vi "最大下移距离.vi"(9 "偏移量":cluster{"X":i32, "Y":i32}, 10 "数组 2":u32[][](array[colorbox]), 11 "数组":u32[][](array[colorbox])) -> (3 "最大下移距离":i32)   [LabVIEW 2012]
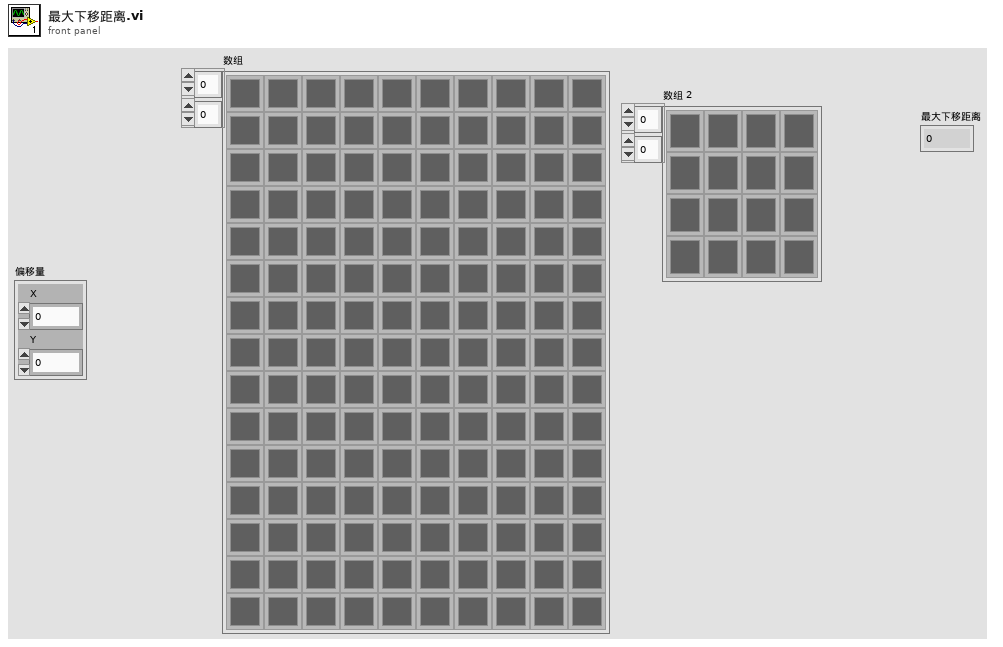
[diagram p1: front panel]
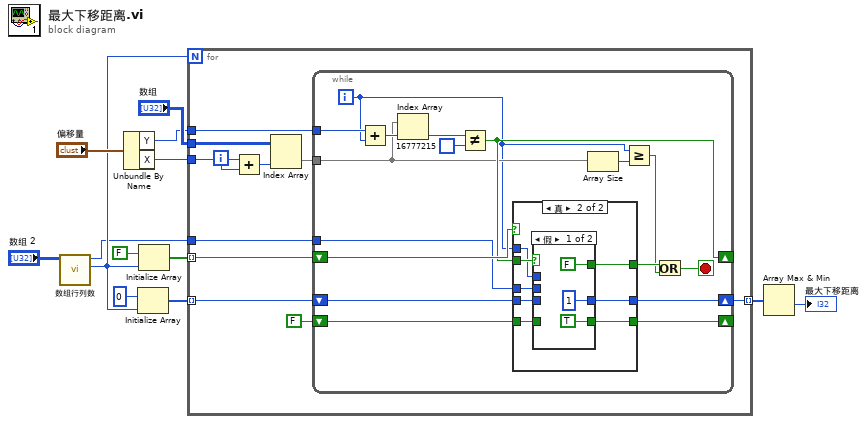
[diagram p0: block diagram]
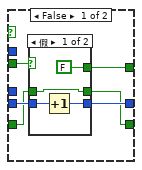
[diagram p2: hidden frame]
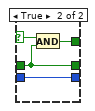
[diagram p3: hidden frame]
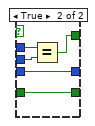
[diagram p4: hidden frame]
diagram:
  n1 = call "数组行列数.vi"("数组"="数组 2") -> ("列"=w2:i32, "行"=w1:i32)  [unwired: 9 in]
  n2 = Unbundle By Name("偏移量") -> ("Y"=w6:i32, "X"=w5:i32)
  n3 = Initialize Array(0, w2) -> (w9:i32[])
  n4 = Initialize Array(FALSE, w2) -> (w10:bool[])
  n5 = for {
    N: w2 -> [_]
    tunnel: "数组" -> [w24]
    tunnel: w6 -> [w17]
    tunnel: w5 -> [w23]
    tunnel: w10 -> [w19] mode=indexing
    tunnel: w9 -> [w18] mode=indexing
    tunnel: [w16] -> w8 mode=indexing
    tunnel: w1 -> [w14]
    i -> [w22]
    n6 = Add(x=w23, y=w22) -> (x+y=w21:i32)
    n7 = Index Array(array=w24, index (col)=w21) -> (element=w20:u32[])  [unwired: 1 in]
    n8 = while {
      tunnel: w20 -> [w31]
      shift-right: [w36] -> _
      shift-left: w19 -> [w37]
      shift-right: [w34] -> w16
      shift-left: w18 -> [w35]
      tunnel: w17 -> [w41]
      shift-right: [w32] -> _
      shift-left: FALSE -> [w33]
      tunnel: w14 -> [w25]
      i -> [w26]
      stop <- w27 stop-if-true
      n9 = Add(x=w41, y=w26) -> (x+y=w40:i32)
      n10 = Index Array(array=w31, index=w40) -> (element=w39:u32)
      n11 = Not Equal?(x=w39, y=u32 16777215) -> (x != y?=w36:bool)
      n12 = case shown="真" w37 {
        tunnel: w36 -> [w47 w63]
        tunnel: w35 -> [w46 w62]
        tunnel: [w45 w61] -> w34
        tunnel: w33 -> [w44 w60]
        tunnel: [w43 w59] -> w32
        tunnel: [w42 w56] -> w29
        tunnel: w26 -> [_ w57]
        tunnel: w25 -> [_ w58]
        frame False {
          n13 = case shown="假" w47 {
            selector: w47 -> [_ w54]
            tunnel: [w50 w55] -> w45
            tunnel: w46 -> [w51 w55]
            tunnel: w44 -> [w49 w53]
            tunnel: [w49 w53] -> w43
            tunnel: [FALSE w52] -> w42
            frame False {
              n14 = Increment(x=w51) -> (x+1=w50:i32)
            }
            frame True {
              n15 = And(x=w54, y=w53) -> (x .and. y?=w52:bool)
            }
          }
        }
        frame True {
          n16 = case shown="假" w63 {
            tunnel: w62 -> [_ w71]
            tunnel: [1 w71] -> w61
            tunnel: w60 -> [_ w70]
            tunnel: [TRUE w70] -> w59
            tunnel: w58 -> [_ w69]
            tunnel: w57 -> [_ w68]
            tunnel: [FALSE w67] -> w56
            frame False {
            }
            frame True {
              n17 = Equal?(x=w68, y=w69) -> (x = y?=w67:bool)
            }
          }
        }
      }
      n18 = Array Size(array=w31) -> (size(s)=w30:i32)
      n19 = Greater Or Equal?(x=w26, y=w30) -> (x >= y?=w28:bool)
      n20 = Or(x=w29, y=w28) -> (x .or. y?=w27:bool)
    }
  }
  n21 = Array Max & Min(array=w8) -> (min value=→"最大下移距离":i32)  [unwired: 3 out]
